vi "Read mRoomVec.vi"(8 "error in (no error)":errorcluster, 11 "Maze":refnum<class "Maze.lvclass">) -> (0 "error out":errorcluster, 2 "mRoomVec":refnum<class "Room.lvclass">[](array[class]), 3 "Maze":refnum<class "Maze.lvclass">)   [LabVIEW 2020, in "Maze.lvclass"]
uses:
  Maze.lvclass
  ConcreteMazeSite/Room/Room.lvclass
  Maze.lvclass/Maze.ctl
  TypeDef/privateDataDVR.ctl
  TypeDef/privateData.ctl
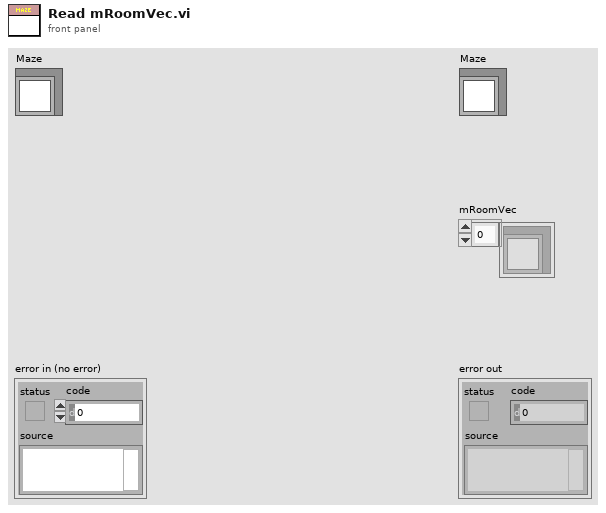
[diagram p1: front panel]
types:
  T1 = typedef "Maze.lvclass/privateDataDVR.ctl" = refnum<data-value>
  T2 = typedef "Maze.lvclass/privateData.ctl" = cluster{"mRoomVec":refnum<class "Room.lvclass">[]}
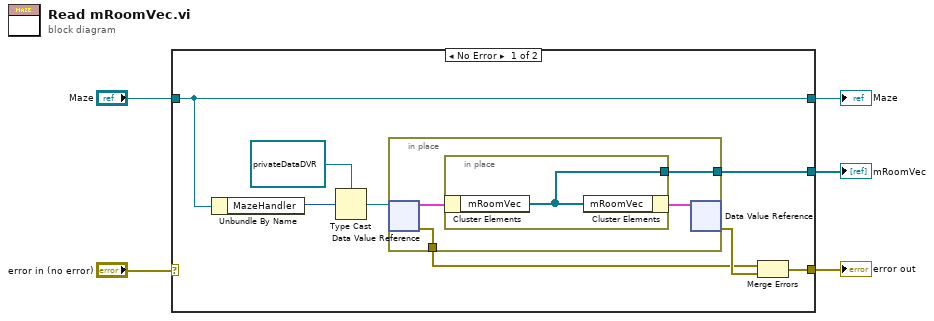
[diagram p0: block diagram]
diagram:
  n1 = case shown="No Error" "error in (no error)" {
    selector: "error in (no error)" -> [_ w19]
    tunnel: "Maze" -> [w9 w20]
    tunnel: [w9 w20] -> w4
    tunnel: [w8 w19] -> w3
    tunnel: [w6 _] -> w1
    frame No Error {
      n2 = Unbundle By Name(w9) -> ("MazeHandler"=w11:u32)
      n3 = Type Cast(type=T1 refnum ("privateDataDVR"), x=w11) -> (*(type *) &x=w13:T1)
      n4 = in-place {
        in-place-border: [w16] -> w10
        in-place-border: [w14] -> w6
        n5 = in-place-dvr #1(w13) -> (w17:T2, w16:errorcluster)
        n6 = in-place {
          in-place-border: [w18] -> w14
          n7 = in-place-cluster #2(w17) -> ("mRoomVec"=w18:refnum<class "Room.lvclass">[])
          n8 = in-place-cluster #2("mRoomVec"=w18) -> (w15:T2)
        }
        n9 = in-place-dvr #1(w15) -> (w12:errorcluster)  [unwired: 1 out]
      }
      n10 = Merge Errors(w10, w12) -> (w8:errorcluster)
    }
    frame Error {
    }
  }
  "error out" <- w3
  "Maze" <- w4
  "mRoomVec" <- w1
